vi "Set Active User.vi"   [LabVIEW 2016]
uses:
  <vilib>/addons/_JKI.lib/REST Client/classes/REST Client/HTTP Header.ctl
  <userlib>/_MGI/Application Control/MGI VI Reference/MGI Current VI's Reference.vi
  <vilib>/addons/_JKI.lib/REST Client/classes/REST Client/REST Client.lvclass
panel:
  # "When you begin using this machine,\nplease run this VI."
types:
  T1 = enum32{"Invalid", "Standard", "Closed", "Hidden", "Minimized", "Maximized"}
  T2 = enum32{"invalid app kind", "Development System", "Run Time System", "Student Edition", "Embedded LabVIEW", "Evaluation", "Custom"}
  T3 = cluster{"Client ID":string, "Client Secret":string, "Redirect URI":string, "Token Endpoint":string, "Scope":string}
  T4 = enum16{"Rainbow 2", "THz 1", "Home-built Ti:S laser", "JEOL AFM", "Cypher", "Agilent AFM", "Montana Cryostat", "MFP3D", "PPMS2", "Nanosurf Easyscan 2/Portable", "PPMS", "Oxford DR200", "Leiden CF", "Leiden MNK"}
  T5 = typedef "REST Client.lvlib/REST Client.lvclass/HTTP Header.ctl" = cluster{"header":string, "value":string}
  T6 = cluster{"Core":cluster{"Current VI Reference":refnum<vi>, "Close Panel on Exit?":bool}, "Authorization":T5[], "Refresh Token":string, "Auth Timeout":dbl, "Users":cluster{"gid":string[], "names":string[]}, "Machine GID":string, "Machine Name":string, "User GID":string, "Date/Time":string}
  T7 = cluster{"Current VI Reference":refnum<vi>, "Close Panel on Exit?":bool}
  T8 = cluster{"id":i32, "gid":string, "resource_type":string, "name":string}[]
  T9 = cluster{"id":i32, "gid":string, "name":string, "resource_type":string}[]
  T10 = cluster{"Array":cluster{"id":i32, "gid":string, "resource_type":string, "user":cluster{"id":i32, "gid":string, "resource_type":string, "name":string}}[]}
  T11 = cluster{"id":i32, "gid":string, "resource_type":string, "user":cluster{"id":i32, "gid":string, "resource_type":string, "name":string}}[]
  T12 = cluster{"id":i32, "gid":string, "resource_type":string, "name":string}
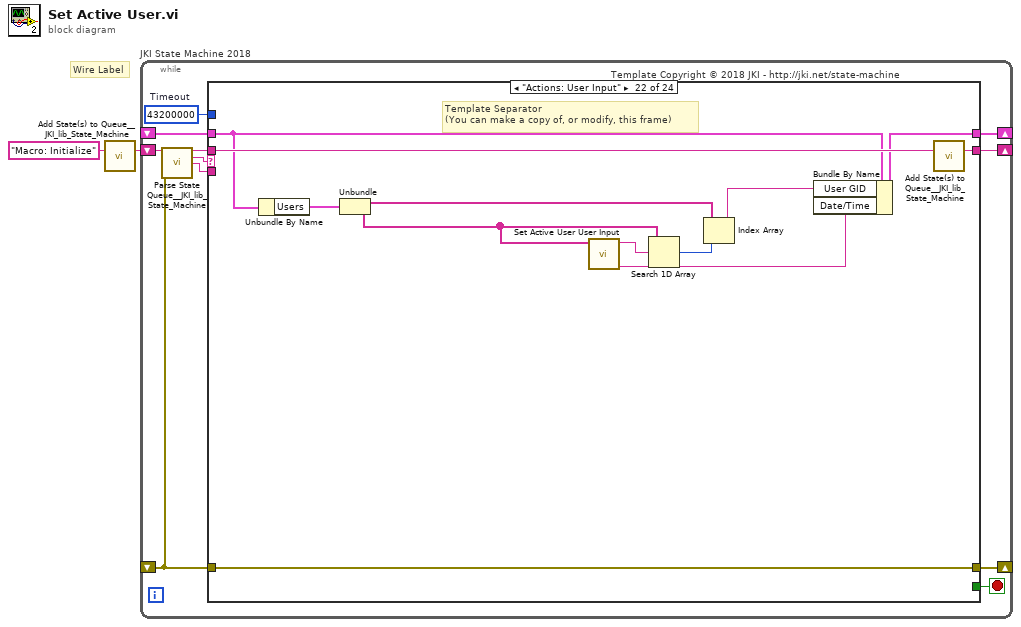
[diagram p0: block diagram]
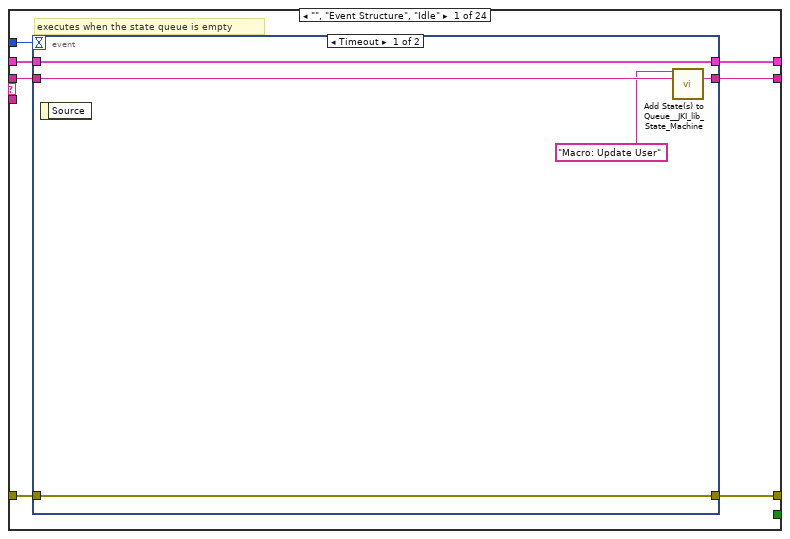
[diagram p2: hidden frame]
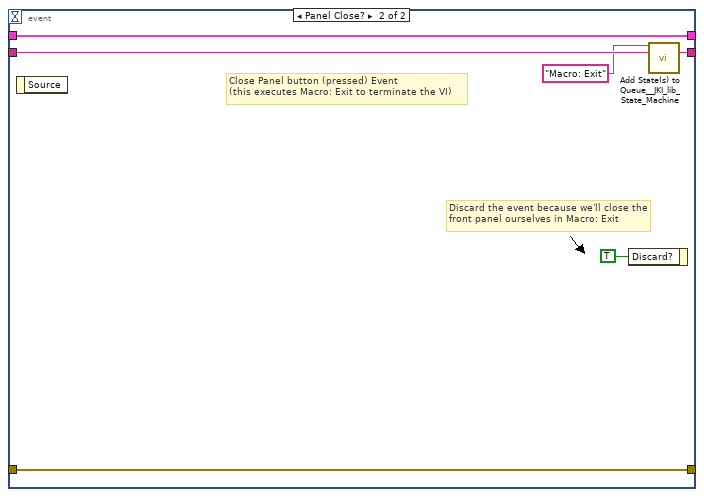
[diagram p3: hidden frame]
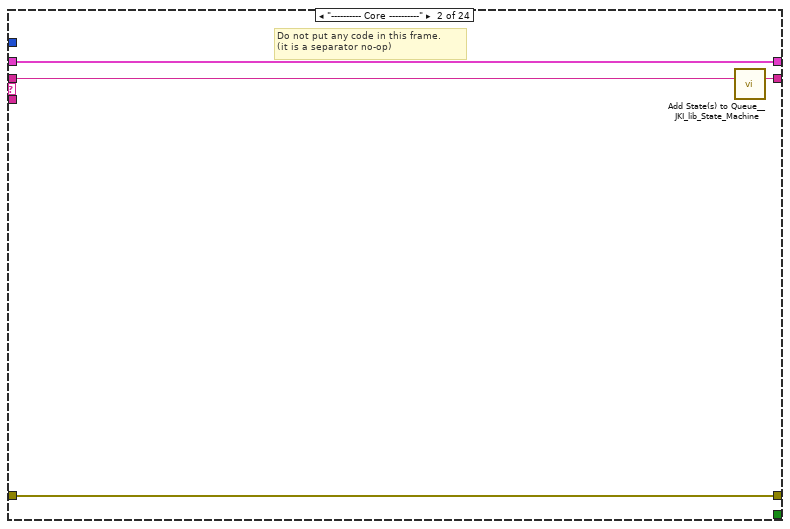
[diagram p4: hidden frame]
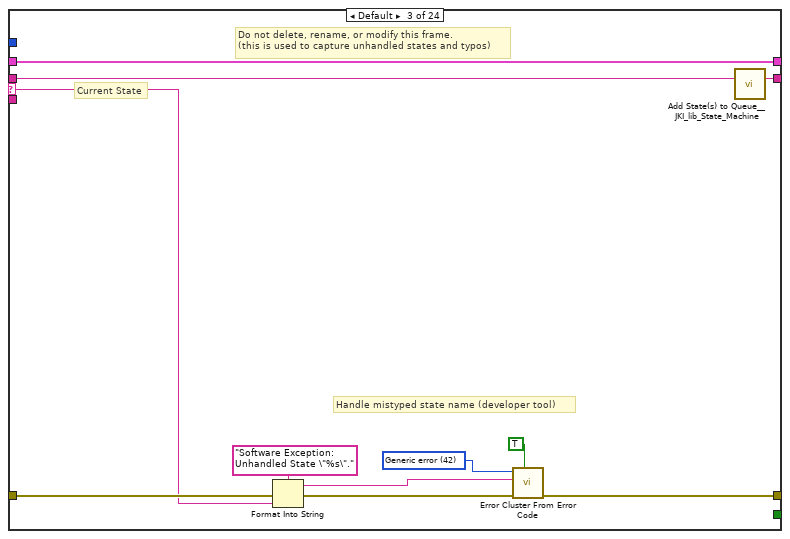
[diagram p5: hidden frame]
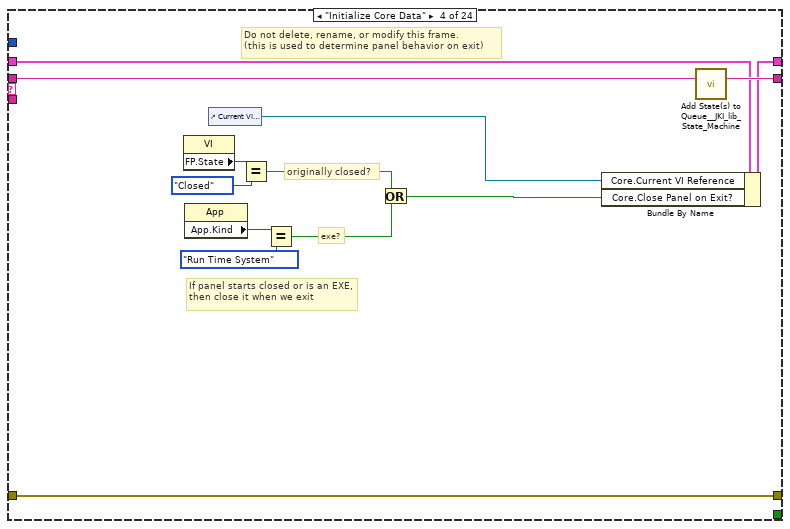
[diagram p6: hidden frame]
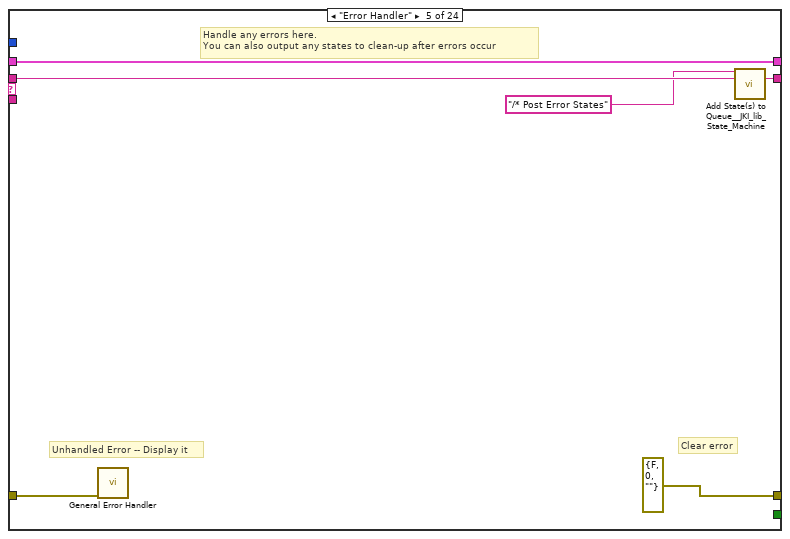
[diagram p7: hidden frame]
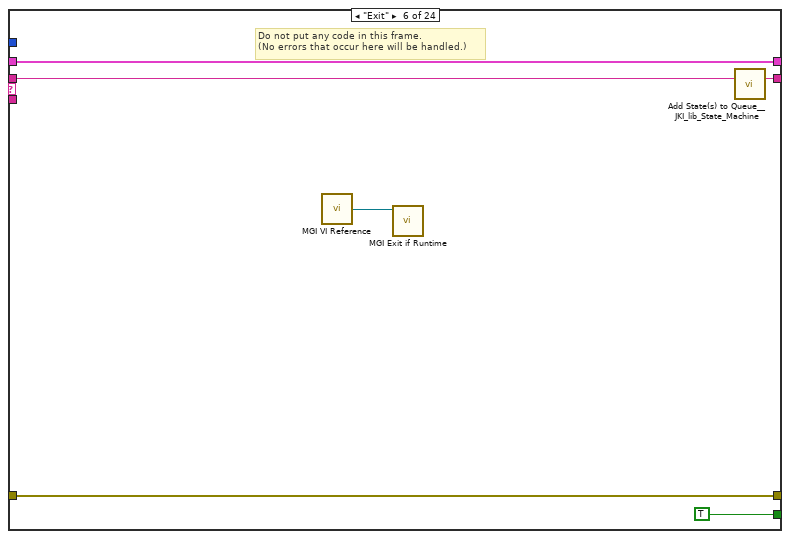
[diagram p8: hidden frame]
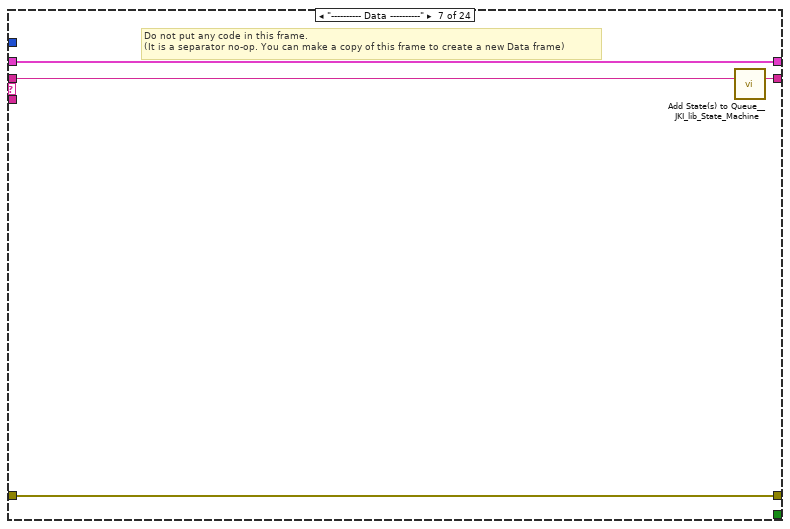
[diagram p9: hidden frame]
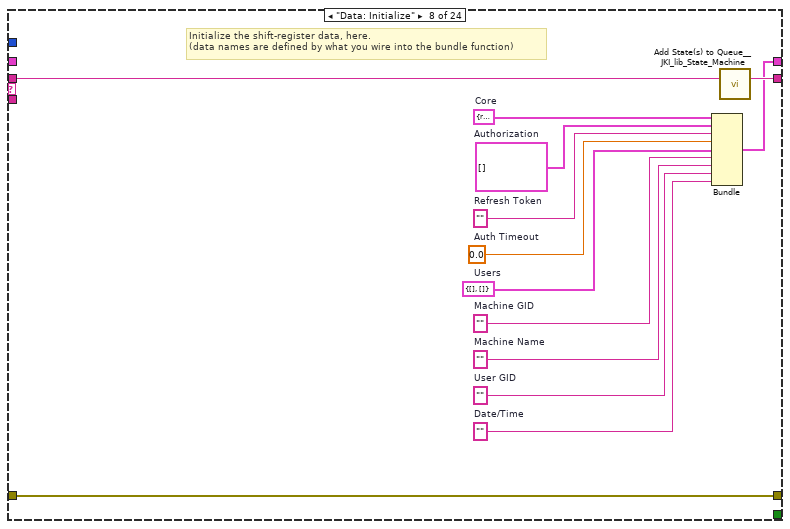
[diagram p10: hidden frame]
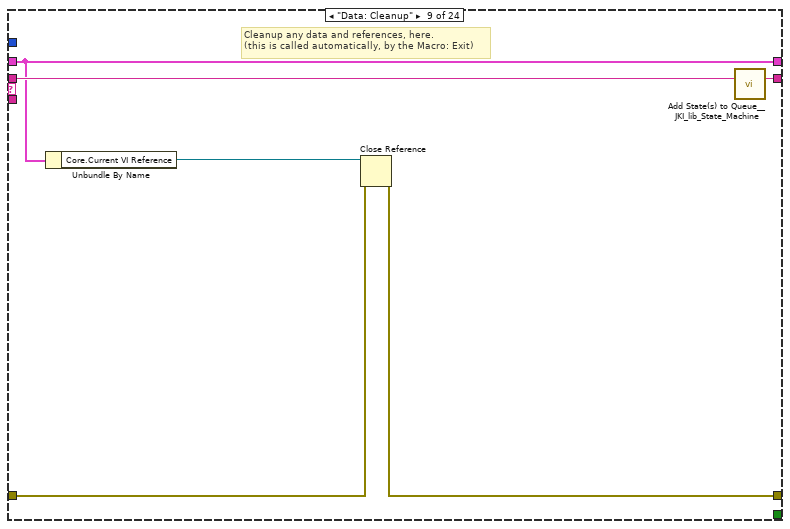
[diagram p11: hidden frame]
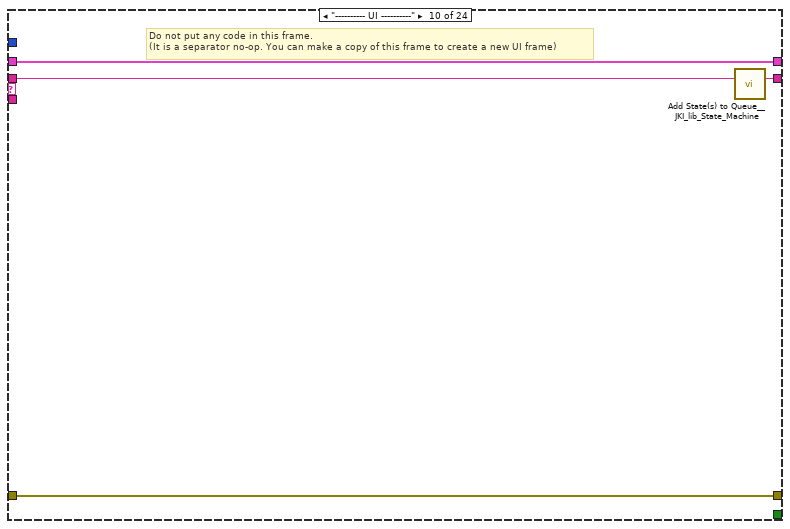
[diagram p12: hidden frame]
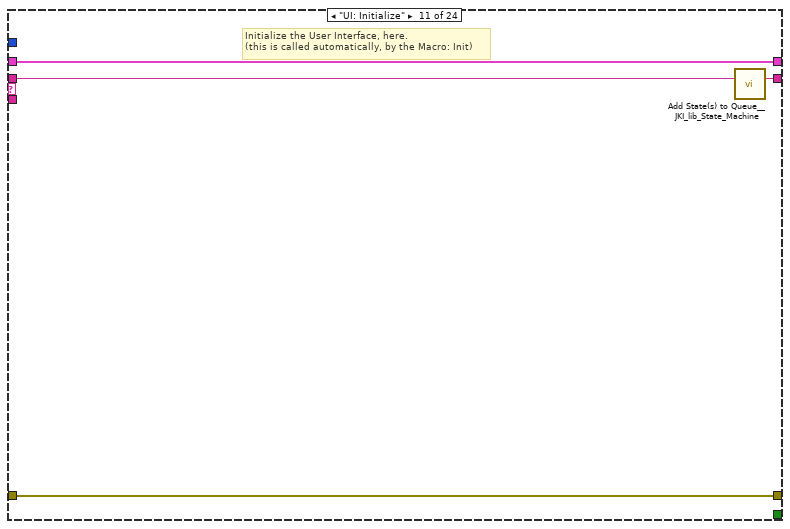
[diagram p13: hidden frame]
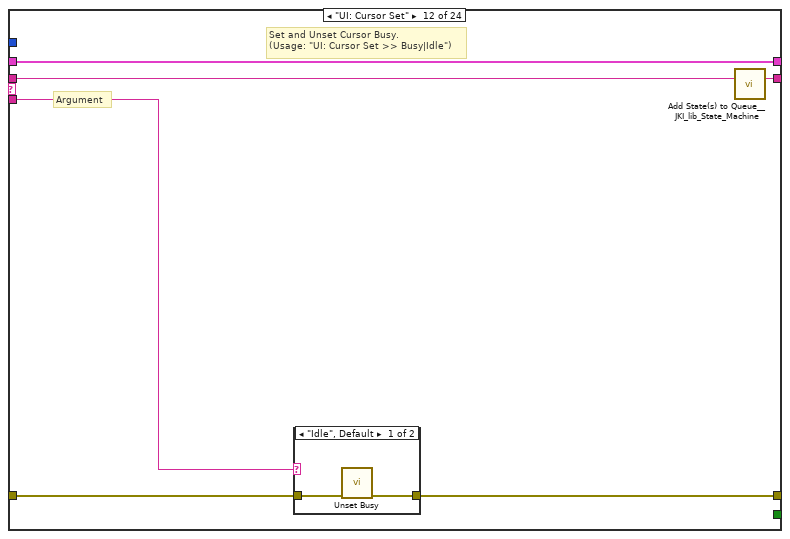
[diagram p14: hidden frame]
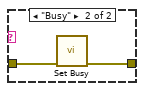
[diagram p15: hidden frame]
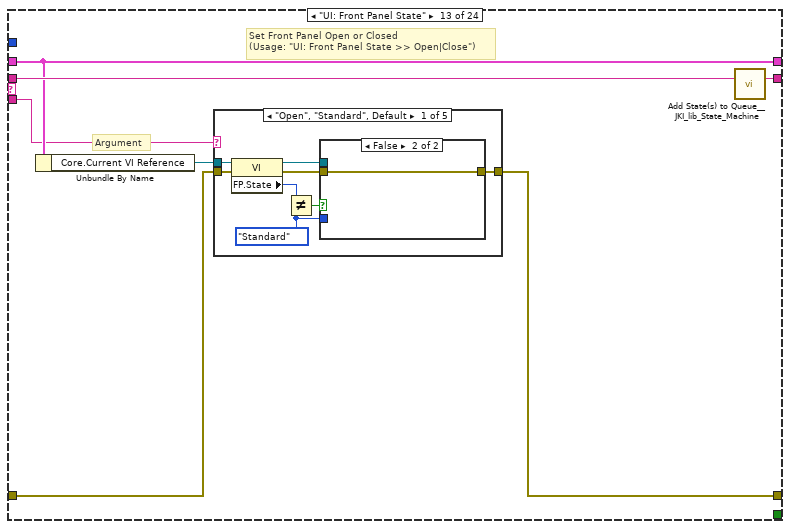
[diagram p16: hidden frame]
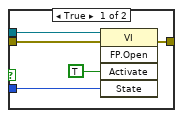
[diagram p17: hidden frame]
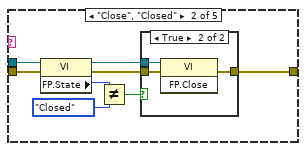
[diagram p18: hidden frame]
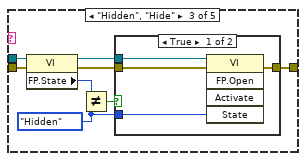
[diagram p20: hidden frame]
diagram:
  # "Wire Label"
  n1 = call <vilib>:"Add State(s) to Queue__JKI_lib_State_Machine.vi"("State(s) in (\"\")"="Macro: Initialize") -> ("States Out"=w2:string)  [unwired: 14 in]
  n2 = while "JKI State Machine 2018" {
    shift-right: [w6] -> _
    shift-left: _ -> [w5]
    shift-right: [w9] -> _
    shift-left: _ -> [w3]
    shift-right: [w8] -> _
    shift-left: w2 -> [w10]
    stop <- w7 stop-if-true
    w4 = 43200000  # Timeout
    # "Template Copyright © 2018 JKI - http://jki.net/state-machine"
    n3 = call <vilib>:"Parse State Queue__JKI_lib_State_Machine.vi"("State Queue"=w10, "Error In (no error)"=w3) -> ("Remaining States"=w12:string, "Current State"=w13:string, "Arguments"=w11:string)  [unwired: 11 in]
    n4 = case shown="\"Actions: User Input\"" w13 {
      selector: w13 -> [_ _ w36 _ _ _ _ _ _ _ _ _ _ _ _ _ _ _ _ _ _ _ _ _]
      tunnel: w12 -> [w20 w35 w40 w59 w65 w71 w75 w88 w94 w98 w102 w108 w119 w188 w193 w198 w208 w212 w227 w242 w259 w274 w294 w322]
      tunnel: w11 -> [_ _ _ _ _ _ _ _ _ _ _ w103 w113 _ _ _ _ _ _ _ _ _ _ _]
      tunnel: w5 -> [w18 w32 w38 w52 w62 w69 w72 _ w89 w95 w100 w106 w115 w185 w190 w195 w205 w209 w224 w239 w248 w272 w279 w320]
      tunnel: [w17 w33 w42 w56 errorcluster {"status"=FALSE, "code"=0, "source"=""} ("error out") w68 w73 w85 w90 w96 w99 w104 w116 w186 w191 w196 w206 w210 w213 w240 w243 w267 w285 w315] -> w9
      tunnel: w3 -> [w16 w33 w41 w56 w61 w68 w73 w85 w91 w96 w99 w105 w117 w186 w191 w196 w206 w210 w214 w240 w249 w267 w276 w305]
      tunnel: [w19 w34 w39 w58 w64 w70 w74 w87 w93 w97 w101 w107 w118 w187 w192 w197 w207 w211 w226 w241 w258 w273 w293 w321] -> w8
      tunnel: [_ _ _ _ _ TRUE _ _ _ _ _ _ _ _ _ _ _ _ _ _ _ _ _ _] -> w7
      tunnel: [w15 w32 w38 w57 w62 w69 w72 w86 w89 w95 w100 w106 w115 w185 w190 w195 w205 w209 w223 w239 w247 w271 w278 w320] -> w6
      tunnel: w4 -> [w14 _ _ _ _ _ _ _ _ _ _ _ _ _ _ _ _ _ _ _ _ _ _ _]
      frame "", "Event Structure", "Idle" {
        # "executes when the state queue is empty"
        n5 = event shown="[0] Timeout" {
          selector: _ -> [_ _]
          dyn-events: _ -> [_ _]
          timeout: w14 -> [_ _]
          tunnel: w20 -> [w25 w31]
          tunnel: [w24 w30] -> w19
          tunnel: w18 -> [w22 w28]
          tunnel: [w23 w29] -> w17
          tunnel: w16 -> [w23 w29]
          tunnel: [w22 w28] -> w15
          event Timeout {
            n6 = event-data() -> ()  [unwired: 1 in, 1 out]
            n7 = call <vilib>:"Add State(s) to Queue__JKI_lib_State_Machine.vi"("State(s) in Front (\"\")"="Macro: Update User", "State(s) in (\"\")"=w25) -> ("States Out"=w24:string)  [unwired: 13 in]
          }
          event Panel Close? {
            # "Discard the event because we'll close the front panel ourselves in Macro: Exit"
            # "Close Panel button (pressed) Event\n(this executes Macro: Exit to terminate the VI)"
            n8 = event-data() -> ()  [unwired: 1 in, 1 out]
            n9 = event-data("Discard?"=TRUE) -> ()  [unwired: 1 in, 1 out]
            n10 = call <vilib>:"Add State(s) to Queue__JKI_lib_State_Machine.vi"("State(s) in Front (\"\")"="Macro: Exit", "State(s) in (\"\")"=w31) -> ("States Out"=w30:string)  [unwired: 13 in]
          }
        }
      }
      frame "---------- Core ----------" {
        # "Do not put any code in this frame.\n(it is a separator no-op)"
        n11 = call <vilib>:"Add State(s) to Queue__JKI_lib_State_Machine.vi"("State(s) in (\"\")"=w35) -> ("States Out"=w34:string)  [unwired: 14 in]
      }
      frame Default {
        w45 = 42 items=["No error", "Argument error", "Memory is full", "Out of zone", "End of file", "File already open", "Generic file I/O error", "File not found", "File permission error", "Disk is full", "Duplicate path", "Too many files open", "System feature not enabled", "Resource file not found", "Cannot add resource", "Resource not found", "Image not found", "Image memory error", "Pen does not exist", "Config type invalid", "Config token not found", "Config parse error", "Config memory error", "Bad external code format", "Bad external code offset", "External code not present", "Null window", "Destroy window error", "Null menu", "Print aborted", "Bad print record", "Print driver error", "Windows error during printing", "Memory error during printing", "Print dialog error", "Generic print error", "Invalid device refnum", "Device not found", "Device parameter error", "Device unit error", "Cannot open device", "Device call aborted", "Generic error", "Cancelled by user", "Object ID too low", "Object ID too high", "Object not in heap", "Unknown heap", "Unknown object (invalid DefProc)", "Unknown object (DefProc not in table)", "Message out of range", "Invalid (null) method", "Unknown message", "Manager call not supported", "Bad address", "Network operation in progress", "Network operation timed out", "Connection is busy", "Network attribute not supported", "Network error", "Address in use", "System out of memory", "Connection aborted", "Connection refused", "Not connected", "Already connected", "Connection closed", "Initialization error (interapplication manager)", "Bad occurrence", "Wait on unbound occurrence handler", "Occurrence queue overflow", "Datalog type conflict", "Unused", "Unrecognized type (interapplication manager)", "Memory corrupt", "Failed to make temporary DLL", "Old CIN version", "Drag socket not found", "Failed to load drop-object", "Failed to register OLE object", "Failed to release OLE object", "Format specifier type mismatch", "Unknown format specifier", "Too few format specifiers", "Too many format specifiers", "Scan failed", "Newer CIN version", "Error converting to variant", "Runtime menu error", "Password tampered", "Variant attribute not found", "Incompatible variant data type", "Event data is not available", "Event Store is not present", "Occurrence is not found", "Event Queue is not created", "Event info is not available", "Refnum passed is NULL", "Error retrieving Class GUID", "Error retrieving CoClass GUID", "Error retrieving TypeLib GUID.", "Bad built application magic bytes.", "Specific driver is different from the specific driver associated with the Logical Name.", "There is no session opened to the class driver.", "Max Error", "MAX - Error with config objects", "MAX - Error loading configuration", "MAX - Group not supported"]
        # "Current State"
        # "Do not delete, rename, or modify this frame.\n(this is used to capture unhandled states and typos)"
        # "Handle mistyped state name (developer tool)"
        n12 = Format Into String(format string="Software Exception: Unhandled State \"%s\"." ("message"), error in=w41, w36) -> (resulting string=w44:string, error out=w43:errorcluster)  [unwired: 1 in]
        n13 = call <vilib>:"Error Cluster From Error Code.vi"("show call chain? (False)"=TRUE, "error in (no error)"=w43, "error message (\"\")"=w44, "error code (0)"=w45) -> ("error out"=w42:errorcluster)  [unwired: 5 in]
        n14 = call <vilib>:"Add State(s) to Queue__JKI_lib_State_Machine.vi"("State(s) in (\"\")"=w40) -> ("States Out"=w39:string)  [unwired: 14 in]
      }
      frame "Initialize Core Data" {
        # "Do not delete, rename, or modify this frame.\n(this is used to determine panel behavior on exit)"
        # "originally closed?"
        # "exe?"
        # "If panel starts closed or is an EXE, then close it when we exit"
        n15 = property class="VI"() -> ("FP.State"=w49:T1)  [unwired: 2 in, 2 out]
        n16 = property class="App"() -> ("App.Kind"=w55:T2)  [unwired: 2 in, 2 out]
        n17 = control-ref of="Current VI Reference"() -> (w50:refnum<vi>)
        n18 = Equal?(x=w49, y=T1."Closed" ("Front Panel Window:State")) -> (x = y?=w47:bool)
        n19 = Equal?(x=w55, y=T2."Run Time System" ("Application:Kind")) -> (x = y?=w53:bool)
        n20 = Or(x=w47, y=w53) -> (x .or. y?=w51:bool)
        n21 = Bundle By Name(cluster=w52, "Core.Current VI Reference"=w50, "Core.Close Panel on Exit?"=w51) -> (w57:T6)
        n22 = call <vilib>:"Add State(s) to Queue__JKI_lib_State_Machine.vi"("State(s) in (\"\")"=w59) -> ("States Out"=w58:string)  [unwired: 14 in]
      }
      frame "Error Handler" {
        # "Unhandled Error -- Display it"
        # "Handle any errors here.\nYou can also output any states to clean-up after errors occur"
        # "Clear error"
        n23 = call <vilib>:"General Error Handler.vi"("error in (no error)"=w61) -> ()  [unwired: 10 in, 5 out]
        n24 = call <vilib>:"Add State(s) to Queue__JKI_lib_State_Machine.vi"("State(s) in Front (\"\")"="/* Post Error States", "State(s) in (\"\")"=w65) -> ("States Out"=w64:string)  [unwired: 13 in]
      }
      frame "Exit" {
        # "Do not put any code in this frame.\n(No errors that occur here will be handled.)"
        n25 = call-poly <userlib>:"MGI VI Reference.vi"() -> ("Current VI's Reference"=w66:refnum<vi>)  [unwired: 1 in]
        n26 = call <userlib>:"MGI Exit if Runtime.vi"("VI Reference (Top Level)"=w66) -> ()  [unwired: 11 in]
        n27 = call <vilib>:"Add State(s) to Queue__JKI_lib_State_Machine.vi"("State(s) in (\"\")"=w71) -> ("States Out"=w70:string)  [unwired: 14 in]
      }
      frame "---------- Data ----------" {
        # "Do not put any code in this frame.\n(It is a separator no-op. You can make a copy of this frame to create a new Data frame)"
        n28 = call <vilib>:"Add State(s) to Queue__JKI_lib_State_Machine.vi"("State(s) in (\"\")"=w75) -> ("States Out"=w74:string)  [unwired: 14 in]
      }
      frame "Data: Initialize" {
        w76 = cluster{"gid":string[], "names":string[]} {"gid"=[], "names"=[]}  # Users
        w77 = ""  # User GID
        w78 = ""  # Date/Time
        w79 = ""  # Machine Name
        w80 = ""  # Machine GID
        w81 = 0.0  # Auth Timeout
        w82 = ""  # Refresh Token
        w83 = T5[] []  # Authorization
        w84 = T7 {"Current VI Reference"=refnum, "Close Panel on Exit?"=FALSE}  # Core
        # "Initialize the shift-register data, here.\n(data names are defined by what you wire into the bundle function)"
        n29 = Bundle("Core"=w84, "Authorization"=w83, "Refresh Token"=w82, "Auth Timeout"=w81, "Users"=w76, "Machine GID"=w80, "Machine Name"=w79, "User GID"=w77, "Date/Time"=w78) -> (w86:T6)  [unwired: 1 in]
        n30 = call <vilib>:"Add State(s) to Queue__JKI_lib_State_Machine.vi"("State(s) in (\"\")"=w88) -> ("States Out"=w87:string)  [unwired: 14 in]
      }
      frame "Data: Cleanup" {
        # "Cleanup any data and references, here.\n(this is called automatically, by the Macro: Exit)"
        n31 = Unbundle By Name(w89) -> ("Core.Current VI Reference"=w92:refnum<vi>)
        n32 = Close Reference(reference=w92, error in (no error)=w91) -> (error out=w90:errorcluster)
        n33 = call <vilib>:"Add State(s) to Queue__JKI_lib_State_Machine.vi"("State(s) in (\"\")"=w94) -> ("States Out"=w93:string)  [unwired: 14 in]
      }
      frame "---------- UI ----------" {
        # "Do not put any code in this frame.\n(It is a separator no-op. You can make a copy of this frame to create a new UI frame)"
        n34 = call <vilib>:"Add State(s) to Queue__JKI_lib_State_Machine.vi"("State(s) in (\"\")"=w98) -> ("States Out"=w97:string)  [unwired: 14 in]
      }
      frame "UI: Initialize" {
        # "Initialize the User Interface, here.\n(this is called automatically, by the Macro: Init)"
        n35 = call <vilib>:"Add State(s) to Queue__JKI_lib_State_Machine.vi"("State(s) in (\"\")"=w102) -> ("States Out"=w101:string)  [unwired: 14 in]
      }
      frame "UI: Cursor Set" {
        # "Argument"
        # "Set and Unset Cursor Busy.\n(Usage: \"UI: Cursor Set >> Busy|Idle\")"
        n36 = case shown="\"Idle\", Default" w103 {
          tunnel: w105 -> [w110 w112]
          tunnel: [w109 w111] -> w104
          frame "Idle", Default {
            n37 = call <vilib>:"Unset Busy.vi"("error in (no error)"=w110) -> ("error out"=w109:errorcluster)  [unwired: 10 in]
          }
          frame "Busy" {
            n38 = call <vilib>:"Set Busy.vi"("error in (no error)"=w112) -> ("error out"=w111:errorcluster)  [unwired: 9 in, 1 out]
          }
        }
        n39 = call <vilib>:"Add State(s) to Queue__JKI_lib_State_Machine.vi"("State(s) in (\"\")"=w108) -> ("States Out"=w107:string)  [unwired: 14 in]
      }
      frame "UI: Front Panel State" {
        # "Argument"
        # "Set Front Panel Open or Closed\n(Usage: \"UI: Front Panel State >> Open|Close\")"
        n40 = Unbundle By Name(w115) -> ("Core.Current VI Reference"=w114:refnum<vi>)
        n41 = case shown="\"Open\", \"Standard\", Default" w113 {
          tunnel: w117 -> [w125 w140 w151 w164 w177]
          tunnel: [w127 w141 w153 w166 w179] -> w116
          tunnel: w114 -> [w126 w138 w152 w165 w178]
          frame "Open", "Standard", Default {
            w120 = T1."Standard" ("State")
            n42 = property class="VI"(reference=w126, error in=w125) -> (reference out=w123:refnum<vi>, error out=w124:errorcluster, "FP.State"=w122:T1)
            n43 = Not Equal?(x=w122, y=w120) -> (x != y?=w121:bool)
            n44 = case shown="False" w121 {
              tunnel: [w131 w133] -> w127
              tunnel: w124 -> [w130 w133]
              tunnel: w123 -> [w129 _]
              tunnel: w120 -> [w128 _]
              frame True {
                n45 = invoke class="VI" method="FP.Open"(reference=w129, error in=w130, "Activate"=TRUE, "State"=w128) -> (error out=w131:errorcluster)  [unwired: 1 in, 4 out]
              }
              frame False {
              }
            }
          }
          frame "Close", "Closed" {
            n46 = property class="VI"(reference=w138, error in=w140) -> (reference out=w137:refnum<vi>, error out=w139:errorcluster, "FP.State"=w135:T1)
            n47 = Not Equal?(x=w135, y=T1."Closed" ("Front Panel Window:State")) -> (x != y?=w134:bool)
            n48 = case shown="True" w134 {
              tunnel: [w142 w145] -> w141
              tunnel: w139 -> [w142 w144]
              tunnel: w137 -> [_ w143]
              frame False {
              }
              frame True {
                n49 = invoke class="VI" method="FP.Close"(reference=w143, error in=w144) -> (error out=w145:errorcluster)  [unwired: 1 in, 2 out]
              }
            }
          }
          frame "Hidden", "Hide" {
            w146 = T1."Hidden" ("State")
            n50 = property class="VI"(reference=w152, error in=w151) -> (reference out=w149:refnum<vi>, error out=w150:errorcluster, "FP.State"=w148:T1)
            n51 = Not Equal?(x=w148, y=w146) -> (x != y?=w147:bool)
            n52 = case shown="True" w147 {
              tunnel: [w157 w158] -> w153
              tunnel: w150 -> [w156 w158]
              tunnel: w149 -> [w155 _]
              tunnel: w146 -> [w154 _]
              frame True {
                n53 = invoke class="VI" method="FP.Open"(reference=w155, error in=w156, "State"=w154) -> (error out=w157:errorcluster)  [unwired: 2 in, 4 out]
              }
              frame False {
              }
            }
          }
          frame "Minimize", "Minimized" {
            w159 = T1."Minimized" ("State")
            n54 = property class="VI"(reference=w165, error in=w164) -> (reference out=w162:refnum<vi>, error out=w163:errorcluster, "FP.State"=w161:T1)
            n55 = Not Equal?(x=w161, y=w159) -> (x != y?=w160:bool)
            n56 = case shown="True" w160 {
              tunnel: [w170 w171] -> w166
              tunnel: w163 -> [w169 w171]
              tunnel: w162 -> [w168 _]
              tunnel: w159 -> [w167 _]
              frame True {
                n57 = invoke class="VI" method="FP.Open"(reference=w168, error in=w169, "State"=w167) -> (error out=w170:errorcluster)  [unwired: 2 in, 4 out]
              }
              frame False {
              }
            }
          }
          frame "Maximize", "Maximized" {
            w172 = T1."Maximized" ("State")
            n58 = property class="VI"(reference=w178, error in=w177) -> (reference out=w175:refnum<vi>, error out=w176:errorcluster, "FP.State"=w174:T1)
            n59 = Not Equal?(x=w174, y=w172) -> (x != y?=w173:bool)
            n60 = case shown="True" w173 {
              tunnel: [w183 w184] -> w179
              tunnel: w176 -> [w182 w184]
              tunnel: w175 -> [w181 _]
              tunnel: w172 -> [w180 _]
              frame True {
                n61 = invoke class="VI" method="FP.Open"(reference=w181, error in=w182, "State"=w180) -> (error out=w183:errorcluster)  [unwired: 2 in, 4 out]
              }
              frame False {
              }
            }
          }
        }
        n62 = call <vilib>:"Add State(s) to Queue__JKI_lib_State_Machine.vi"("State(s) in (\"\")"=w119) -> ("States Out"=w118:string)  [unwired: 14 in]
      }
      frame "---------- Macro ----------" {
        # "Do not put any code in this frame.\n(It is a separator no-op. You can make a copy of this frame to create a new Macro frame)"
        n63 = call <vilib>:"Add State(s) to Queue__JKI_lib_State_Machine.vi"("State(s) in (\"\")"=w188) -> ("States Out"=w187:string)  [unwired: 14 in]
      }
      frame "Macro: Initialize" {
        # "Initialization Macro\n(This is called once, when the VI starts)"
        n64 = call <vilib>:"Add State(s) to Queue__JKI_lib_State_Machine.vi"("State(s) in Front (\"\")"="Data: Initialize\nInitialize Core Data\nUI: Initialize\nUI: Front Panel State >> Open\nMacro: Update User", "State(s) in (\"\")"=w193) -> ("States Out"=w192:string)  [unwired: 13 in]
      }
      frame "Macro: Update User" {
        # "Do not put any code in this frame.\n(It is a separator no-op. You can make a copy of this frame to create a new Macro frame)"
        n65 = call <vilib>:"Add State(s) to Queue__JKI_lib_State_Machine.vi"("State(s) in Front (\"\")"="Authorization: Handle\nActions: Machine Input\nActions: Get Project Members\nActions: User Input\nActions: Update User" ("State(s) in Front (\"\")"), "State(s) in (\"\")"=w198) -> ("States Out"=w197:string)  [unwired: 13 in]
      }
      frame "Macro: Exit" {
        # "Exit Macro\n(This is called once, when the VI exits)"
        n66 = Unbundle By Name(w205) -> ("Core.Close Panel on Exit?"=w204:bool)
        n67 = Select(t="UI: Front Panel State >> Close", s=w204, f="") -> (s? t:f=w201:string)
        n68 = call <vilib>:"Add State(s) to Queue__JKI_lib_State_Machine.vi"("State(s) in (\"\")"=w201, "State(s) at Back (\"\")"="Data: Cleanup\nExit") -> ("States Out"=w199:string)  [unwired: 13 in]
        n69 = call <vilib>:"Add State(s) to Queue__JKI_lib_State_Machine.vi"("State(s) in Front (\"\")"=w199, "State(s) in (\"\")"=w208) -> ("States Out"=w207:string)  [unwired: 13 in]
      }
      frame "---------- Authorization ----------" {
        # "Template Separator\n(You can make a copy of, or modify, this frame)"
        n70 = call <vilib>:"Add State(s) to Queue__JKI_lib_State_Machine.vi"("State(s) in (\"\")"=w212) -> ("States Out"=w211:string)  [unwired: 14 in]
      }
      frame "Authorization: Handle" {
        # "Your code here.\n(You can make a copy of, or modify, this frame)"
        n71 = Unbundle By Name(w224) -> ("Auth Timeout"=w217:dbl, "Refresh Token"=w225:string, "Authorization"=w219:T5[])
        n72 = Get Date/Time In Seconds() -> (seconds since 1Jan1904=w216:timestamp)
        n73 = To Double Precision Float(number=w216) -> (double precision float=w215:dbl)
        n74 = Less Or Equal?(x=w217, y=w215) -> (x <= y?=w218:bool)
        n75 = case shown="True" w218 {
          tunnel: w225 -> [w230 w238]
          tunnel: [w231 w235] -> w222
          tunnel: [w230 w237] -> w221
          tunnel: [w229 w236] -> w220
          tunnel: w217 -> [w231 _]
          tunnel: w219 -> [w229 _]
          tunnel: w214 -> [w228 w233]
          tunnel: [w228 w232] -> w213
          frame False {
          }
          frame True {
            n76 = call <userlib>:"Asana Authentication.vi"("error in (no error)"=w233, "Authentication Info"=T3 {"Client ID"="1108428692000476", "Client Secret"="803bdca1138fccb00921b8f346728904", "Redirect URI"="https://app.asana.com/api/1.0", "Token Endpoint"="https://app.asana.com/-/oauth_token", "Scope"=""}, "Refresh Token In"=w238) -> ("error out"=w232:errorcluster, "Authentication Header"=w236:T5[], "Refresh Token Out"=w237:string, "Timeout"=w235:dbl)  [unwired: 5 in]
          }
        }
        n77 = Bundle By Name(cluster=w224, "Auth Timeout"=w222, "Refresh Token"=w221, "Authorization"=w220) -> (w223:T6)
        n78 = call <vilib>:"Add State(s) to Queue__JKI_lib_State_Machine.vi"("State(s) in (\"\")"=w227) -> ("States Out"=w226:string)  [unwired: 14 in]
      }
      frame "---------- Actions ----------" {
        # "Template Separator\n(You can make a copy of, or modify, this frame)"
        n79 = call <vilib>:"Add State(s) to Queue__JKI_lib_State_Machine.vi"("State(s) in (\"\")"=w242) -> ("States Out"=w241:string)  [unwired: 14 in]
      }
      frame "Actions: Machine Input" {
        # "Template Separator\n(You can make a copy of, or modify, this frame)"
        n80 = Unbundle By Name(w248) -> ("Authorization"=w255:T5[])
        n81 = To Variant(anything=T4."PPMS2") -> (Variant=w256:variant)
        n82 = call <userlib>:"Get Strings from Enum__ogtk.vi"("error in (no error)"=w249, "Enum"=w256) -> ("error out"=w244:errorcluster, "String Value"=w245:string)  [unwired: 6 in, 2 out]
        n83 = call <userlib>:"Get Tasks.vi"("Authorization"=w255, "error in (no error)"=w244, "Project GID"="1128411193296042") -> ("error out"=w243:errorcluster, "Tasks Out"=w253:T8)  [unwired: 7 in]
        n84 = for {
          tunnel: w253 -> [w262] mode=indexing
          tunnel: [w261] -> w252 mode=indexing
          tunnel: [w260] -> w251 mode=indexing
          n85 = Unbundle(w262) -> ("gid"=w260:string, "name"=w261:string)  [unwired: 2 out]
        }
        n86 = Search 1D Array(1D array=w252, element=w245) -> (index of element=w250:i32)  [unwired: 1 in]
        n87 = Index Array(array=w251, index=w250) -> (element=w246:string)
        n88 = Bundle By Name(cluster=w248, "Machine GID"=w246, "Machine Name"=w245) -> (w247:T6)
        n89 = call <vilib>:"Add State(s) to Queue__JKI_lib_State_Machine.vi"("State(s) in (\"\")"=w259) -> ("States Out"=w258:string)  [unwired: 14 in]
      }
      frame "Actions: User Input" {
        # "Template Separator\n(You can make a copy of, or modify, this frame)"
        n90 = Unbundle By Name(w272) -> ("Users"=w266:cluster{"gid":string[], "names":string[]})
        n91 = Unbundle(w266) -> ("gid"=w265:string[], "names"=w264:string[])
        n92 = call "Set Active User User Input.vi"("Users"=w264) -> ("Date/Time"=w269:string, "Selected User"=w263:string)  [unwired: 9 in]
        n93 = Search 1D Array(1D array=w264, element=w263) -> (index of element=w270:i32)  [unwired: 1 in]
        n94 = Index Array(array=w265, index=w270) -> (element=w268:string)
        n95 = Bundle By Name(cluster=w272, "User GID"=w268, "Date/Time"=w269) -> (w271:T6)
        n96 = call <vilib>:"Add State(s) to Queue__JKI_lib_State_Machine.vi"("State(s) in (\"\")"=w274) -> ("States Out"=w273:string)  [unwired: 14 in]
      }
      frame "Actions: Get Project Members" {
        # "Template Separator\n(You can make a copy of, or modify, this frame)"
        n97 = Unbundle By Name(w279) -> ("Authorization"=w277:T5[], "Machine Name"=w292:string)
        n98 = call <userlib>:"Get Projects.vi"("Authorization"=w277, "error in (no error)"=w276, "Team GID"="6623647313143") -> ("error out"=w275:errorcluster, "Projects Out"=w291:T9)  [unwired: 7 in]
        n99 = for {
          tunnel: w291 -> [w301] mode=indexing
          tunnel: [w300] -> w289 mode=indexing
          tunnel: [w299] -> w288 mode=indexing
          n100 = Unbundle(w301) -> ("gid"=w299:string, "name"=w300:string)  [unwired: 2 out]
        }
        n101 = Search 1D Array(1D array=w289, element=w292) -> (index of element=w287:i32)  [unwired: 1 in]
        n102 = Index Array(array=w288, index=w287) -> (element=w286:string)
        n103 = call <userlib>:"Get Project Members.vi"("Authorization"=w277, "error in (no error)"=w275, "Project GID"=w286) -> ("error out"=w285:errorcluster, "Memberships Out"=w284:T10)  [unwired: 7 in]
        n104 = Unbundle(w284) -> ("Array"=w283:T11)
        n105 = for {
          tunnel: w283 -> [w298] mode=indexing
          tunnel: [w296] -> w282 mode=indexing
          tunnel: [w295] -> w281 mode=indexing
          n106 = Unbundle(w298) -> ("user"=w297:T12)  [unwired: 3 out]
          n107 = Unbundle(w297) -> ("gid"=w296:string, "name"=w295:string)  [unwired: 2 out]
        }
        n108 = Bundle(w282, w281) -> (w280:cluster{string[], string[]})  [unwired: 1 in]
        n109 = Bundle By Name(cluster=w279, "Users"=w280) -> (w278:T6)
        n110 = call <vilib>:"Add State(s) to Queue__JKI_lib_State_Machine.vi"("State(s) in (\"\")"=w294) -> ("States Out"=w293:string)  [unwired: 14 in]
      }
      frame "Actions: Update User" {
        # "Your code here.\n(You can make a copy of, or modify, this frame)"
        n111 = Unbundle By Name(w320) -> ("User GID"=w303:string, "Machine GID"=w304:string, "Authorization"=w307:T5[], "Date/Time"=w302:string)
        n112 = Concatenate Strings("{\"data\": {\"notes\": \"Updated " ("string"), w302, "\", \"assignee\": \"" ("string"), w303, "\"}}" ("string")) -> (w308:string)
        n113 = Concatenate Strings("/tasks/" ("string"), w304) -> (w314:string)
        n114 = call <vilib>:"Create REST Client.vi"("error in (no error)"=w305, "Base URL"="https://app.asana.com/api/1.0") -> ("error out"=w317:errorcluster, "REST Client out"=w319:refnum<class "REST Client.lvclass">)  [unwired: 8 in]
        n115 = call-dynamic "HTTP PUT.vi"("request specific headers"=w307, "error in (no error)"=w317, "Request body"=w308, "Path"=w314, "REST Client in"=w319) -> ("error out"=w316:errorcluster, "REST Client out"=w318:refnum<class "REST Client.lvclass">)  [unwired: 1 in, 4 out]
        n116 = call-dynamic "Destroy REST Client.vi"("error in (no error)"=w316, "REST Client in"=w318) -> ("error out"=w315:errorcluster)  [unwired: 9 in]
        n117 = call <vilib>:"Add State(s) to Queue__JKI_lib_State_Machine.vi"("State(s) in Front (\"\")"="Macro: Exit", "State(s) in (\"\")"=w322) -> ("States Out"=w321:string)  [unwired: 13 in]
      }
    }
  }
